vi "Logging Get Names.vi"(1 "Entries":T1[](array[typedef])) -> (0 "Names":string[](array[string]))   [LabVIEW 2012, in "femtoRoboLib.lvlib"]
uses:
  Log Entry.ctl
  Log Value Type.ctl
  Log Value Cluster.ctl
  femtoRoboLib.lvlib
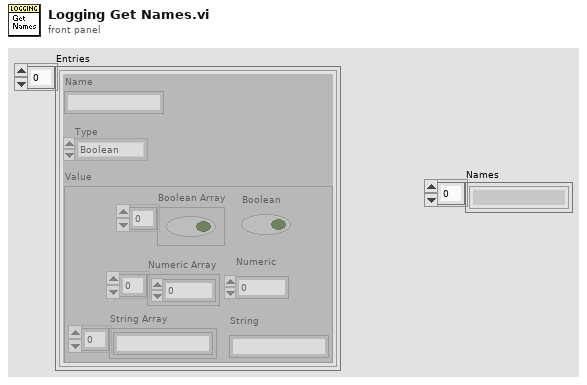
[diagram p1: front panel]
types:
  T1 = typedef "femtoRoboLib.lvlib/Log Entry.ctl" = cluster{"Name":string, "Type":T2, "Value":T3}
  T2 = typedef "femtoRoboLib.lvlib/Log Value Type.ctl" = enum16{"Boolean", "Numeric", "String", "Boolean Array", "Numeric Array", "String Array"}
  T3 = typedef "femtoRoboLib.lvlib/Log Value Cluster.ctl" = cluster{"Boolean Array":bool[], "Boolean":bool, "Numeric Array":dbl[], "Numeric":dbl, "String Array":string[], "String":string}
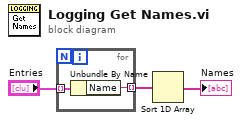
[diagram p0: block diagram]
diagram:
  n1 = for {
    tunnel: "Entries" -> [w5] mode=indexing
    tunnel: [w4] -> w3 mode=indexing
    n2 = Unbundle By Name(w5) -> ("Name"=w4:string)
  }
  n3 = Sort 1D Array(array=w3) -> (sorted array=→"Names":string[])
